vi "Handle Errors.vi"(8 "error in (no error)":errorcluster, 10 "Location":string, 11 "Error Handler Interface In":refnum<class "Error Handler Interface.lvclass">) -> (0 "error out":errorcluster, 3 "Error Handler Interface Out":refnum<class "Error Handler Interface.lvclass">)   [LabVIEW 2020, in "Error Handler Interface.lvclass"]
doc: "The implementation of this VI defines how errors are handled."
uses:
  Error Handler Interface.lvclass
panel:
  out "Error":errorcluster
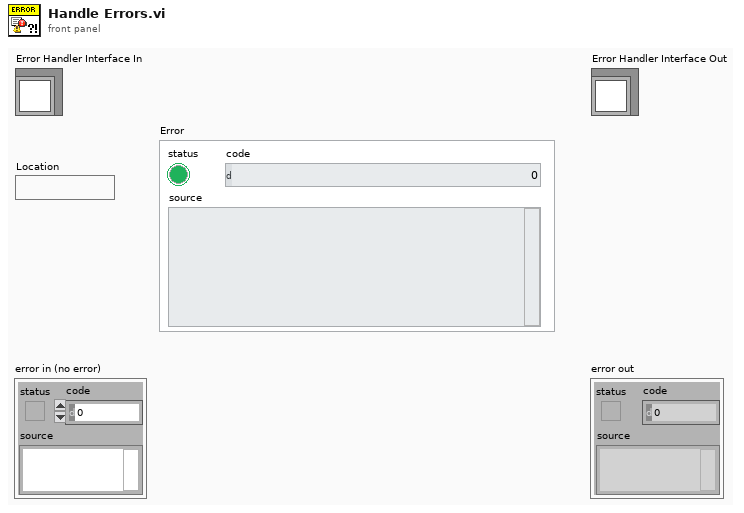
[diagram p1: front panel]
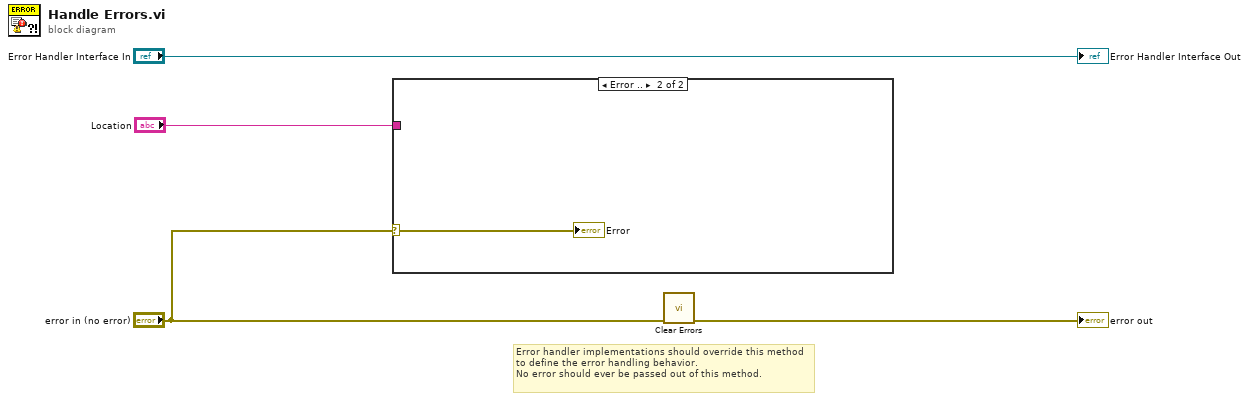
[diagram p0: block diagram]
diagram:
  # "Error handler implementations should override this method to define the error handling behavior. \nNo error should ever be passed out of this method."
  n1 = case shown="Error .." "error in (no error)" {
    selector: "error in (no error)" -> [_ w5]
    tunnel: "Location" -> [_ _]
    frame No Error {
    }
    frame Error {
      "Error" <- w5
    }
  }
  n2 = call <vilib>:"Clear Errors.vi"("error in (no error)"="error in (no error)") -> ("error out"=→"error out":errorcluster)  [unwired: 5 in, 1 out]
  "Error Handler Interface Out" <- "Error Handler Interface In"
